vi "FTW-Regex-ReplaceAll.vi"(0 "String":string, 5 "Search for (Regular Expression)":string, 7 "Replace with":string, 11 "error in":errorcluster) -> (4 "String out":string, 6 "Number of Replacements":i32, 15 "error out":errorcluster)   [LabVIEW 2014]
panel:
  # "Inputs"
  # "Outputs"
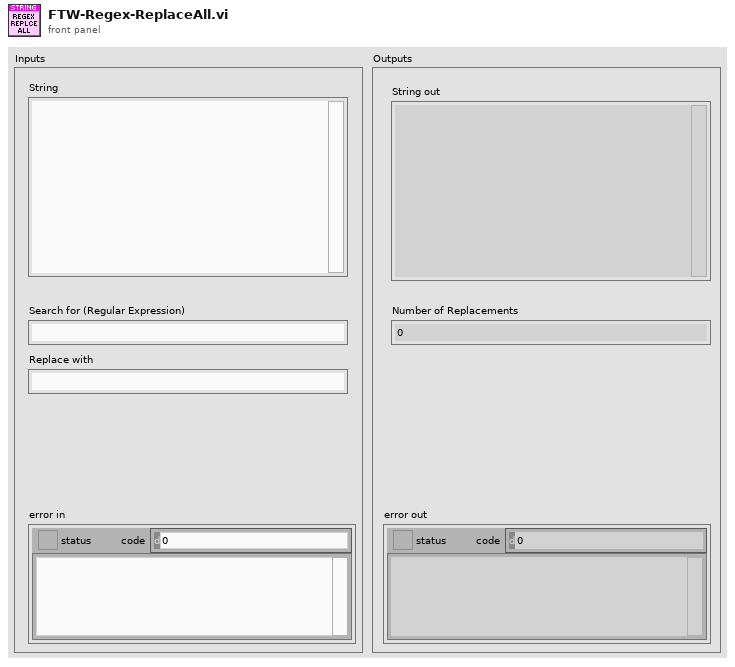
[diagram p1: front panel]
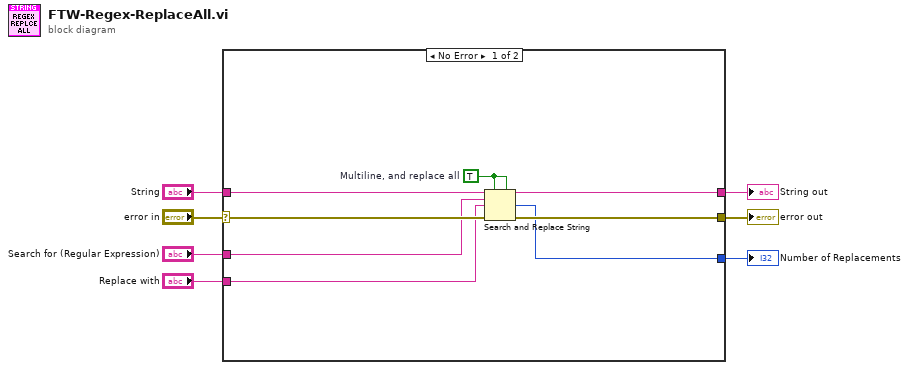
[diagram p0: block diagram]
diagram:
  n1 = case shown="No Error" "error in" {
    selector: "error in" -> [w14 w17]
    tunnel: [w12 w17] -> w7
    tunnel: "String" -> [w15 w16]
    tunnel: [w13 w16] -> w4
    tunnel: "Replace with" -> [w8 _]
    tunnel: [w11 _] -> w3
    tunnel: "Search for (Regular Expression)" -> [w9 _]
    frame No Error {
      w10 = TRUE  # Multiline, and replace all
      n2 = Search and Replace String(replace all?=w10, multiline?=w10, input string=w15, search string=w9, replace string=w8, error in=w14) -> (result string=w13:string, number of replacements=w11:i32, error out=w12:errorcluster)  [unwired: 2 in, 1 out]
    }
    frame Error {
    }
  }
  "error out" <- w7
  "String out" <- w4
  "Number of Replacements" <- w3
